vi "pigeon_ver4_1.vi"() -> ()   [LabVIEW 2017]
uses:
  <vilib>/eio/EIONode/EIONode.xnode
  <vilib>/Platform/TimedLoop/XDataNode/XDataNode.xnode
  <vilib>/Platform/TimedLoop/XDataNode/nitl_modes.ctl
  <vilib>/Platform/TimedLoop/XDataNode/XDNodeRunTimeDep.lvlib
  <vilib>/Platform/TimedLoop/XDataNode/wakeup.ctl
  <vilib>/Platform/TimedLoop/XDataNode/timing_clust.ctl
  <vilib>/rvi/DataTransferAndStorage/Container/XNode/niFpgaContainer.xnode
  <vilib>/rvi/eio/common/nirviEmuTemplateMethod_errors.vi
  <vilib>/rvi/Memory/Memory_Emulation/nirvimemoryFastEmulation.vi
  <vilib>/rvi/Memory/Memory_Emulation/nirvimemoryEmulation.vi
  <vilib>/rvi/interface/RandomDataEmulation/nirviRandomDataFpgaReadWriteTemplate.vi
  <vilib>/rvi/Analysis/common/FxpNativeNode/niFpgaFxpNative.xnode
panel:
  out "ramp loop end?":bool=TRUE
  out "ctr":i16
  out "ramp start val":fxp<+,15,15>
  out "Numeric":i16
  in  "analog ramp on":bool
  out "AI2":i16
  in  "Tab Control":enum32{"pigeon"}(tab)
  in  "AO7_pigeon":i16
  in  "AO7":i16
  in  "AO6":i16
  out "trigger AI1":bool
  in  "Tab Control 2":T1(tab)
  in  "square wave  on?":bool
  in  "square wave period":i32
  in  "IGBTswitch":bool caption="IGBT Switch circular"
  in  "Manual Override":bool
  in  "circular coil current":i16(slide) scale=0.0..32768.0
  in  "analog ramp period":i16
  in  "AO4":bool
  in  "analog wave shape":i16(ring) items=["Triangle", "Sawtooth", "Sin", ""]
  in  "analog ramp on  2":bool
  in  "End Current":fxp<+,16,16>
  out "approx rise time [uSec]":u32
  in  "Update Period (uSec)":u32=500
  in  "Points to Add (2^n - 1)":i16=3
  out "FIFO size":i16
  in  "AO0":i16
  in  "AO1":i16
  in  "AO2":i16
  in  "Run program":bool
  in  "halt processor":bool
  out "control flags":i8 format="%b"
  in  "host operation":i16
  in  "address":u16
  in  "data1":u16
  in  "data2":i32
  in  "repeat program":i32
  out "IP address":i16
  out "PMT1":i16=-4740
  out "ReA":i32
  out "RegB":i16
  out "RegC":i16
  out "exttrigger":bool=TRUE
  out "AI1":i16=161
  out "RegD":i16
  in  "AO4":i16
  in  "AO3":i16
  out "Connector0/AI0":i16
  in  "AO5":i16
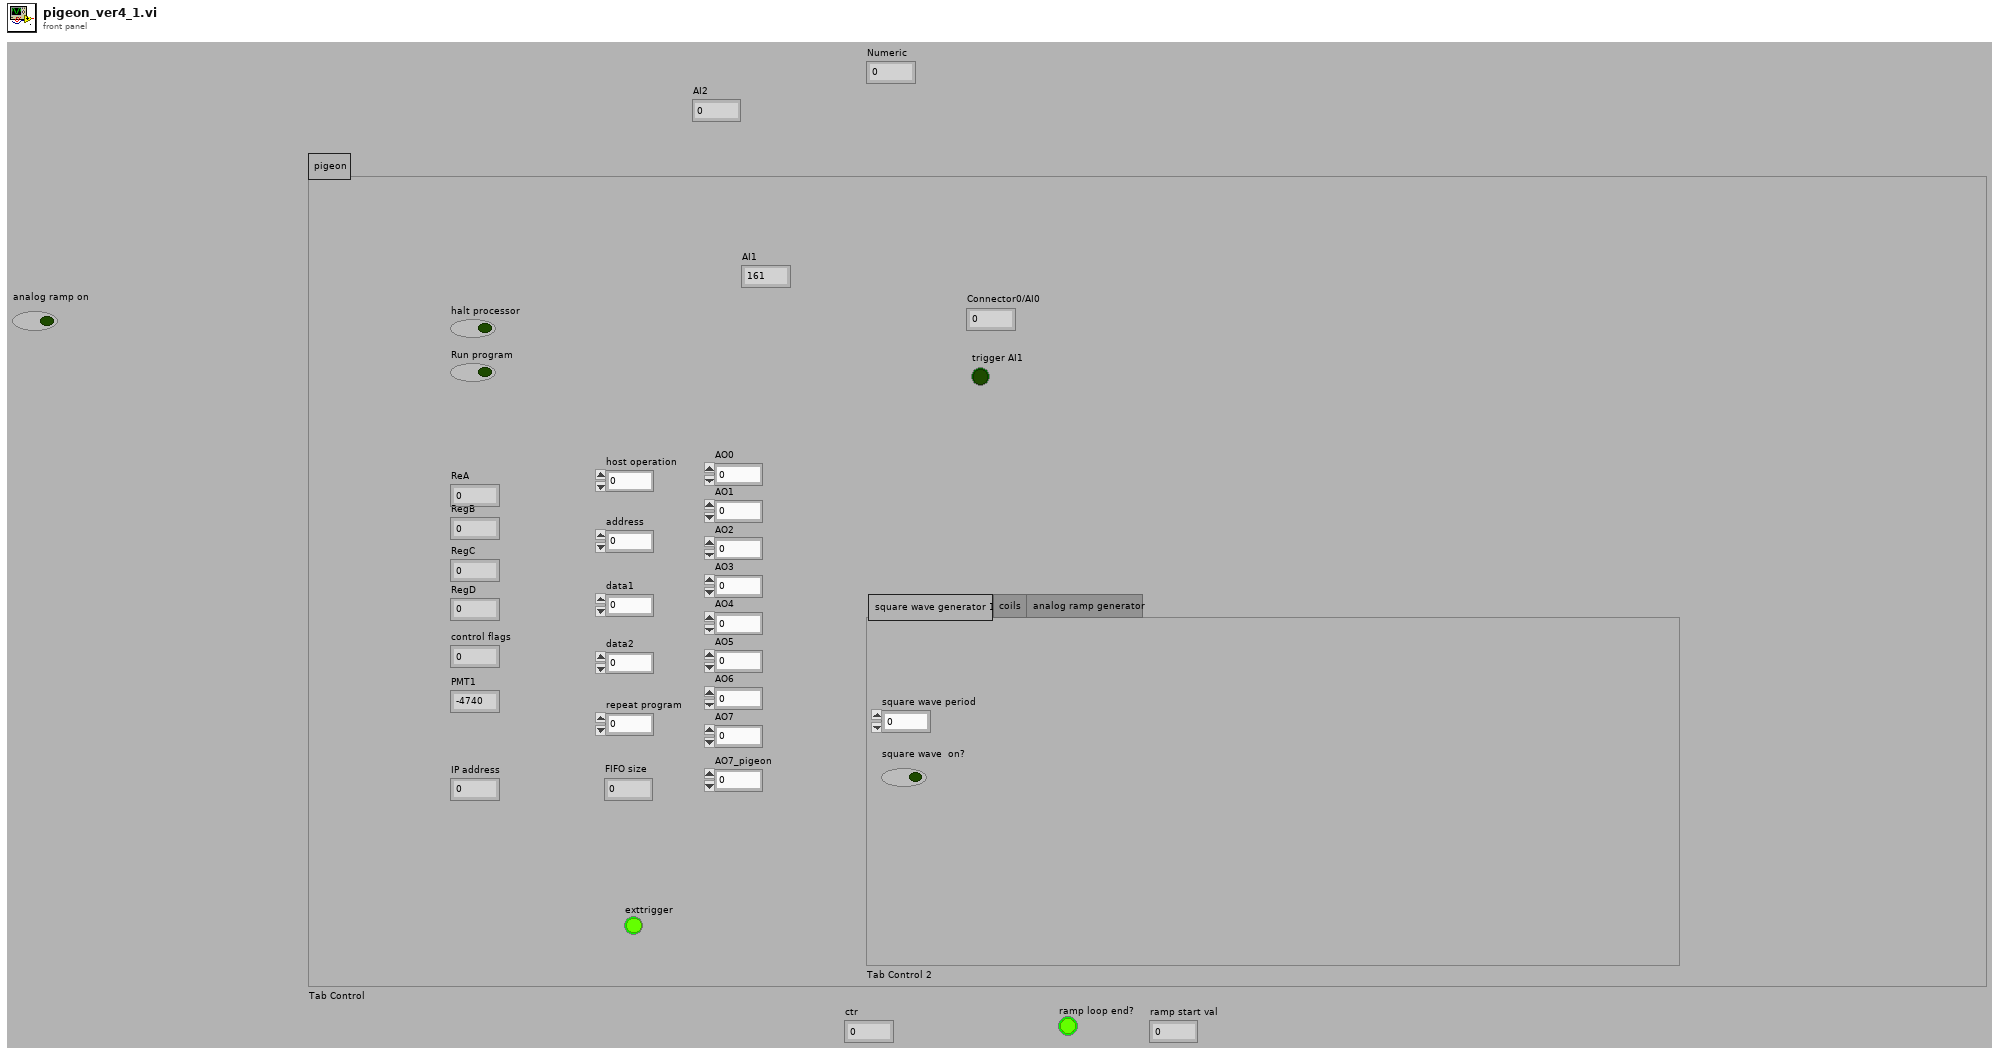
[diagram p1: front panel]
types:
  T1 = enum32{"square wave generator 1", "coils", "analog ramp generator"}
  T2 = typedef "XDNodeRunTimeDep.lvlib/timing_clust.ctl" = cluster{"Expected End [f-1]":u64, "Actual End [f-1]":u64, "Finished Late? [f-1]":bool, "Expected End [i-1]":u64, "Actual End [i-1]":u64, "Finished Late? [i-1]":bool, "Expected Start [i]":u64, "Actual Start [i]":u64, "Expected Start [f]":u64, "Actual Start [f]":u64, "Source Name":string, "Structure Name":string, "Period":i64, "Deadline":i64, "Offset":i64, "Start":i64, "Priority":i32, "Timeout":i32, "Mode":T3, "Wakeup Reason":T4, "Error":errorcluster, "Source Type":string, "Secondary Source Type":string, "Global End Time":u64, "Global Start Time":u64, "Frame Duration":u64, "Iteration Duration":u64, "Assigned CPU":i32, "I/O Scan Engine Mode":u32}
  T3 = typedef "XDNodeRunTimeDep.lvlib/nitl_modes.ctl" = enum32{"No Change", "Process missed periods, maintain original phase", "Discard missed periods, maintain original phase", "Process missed periods, ignore original phase", "Discard missed periods, ignore original phase"}
  T4 = typedef "XDNodeRunTimeDep.lvlib/wakeup.ctl" = enum32{"Normal", "Aborted", "Asynchronous wakeup", "Timing source error", "Timed loop error", "Timeout"}
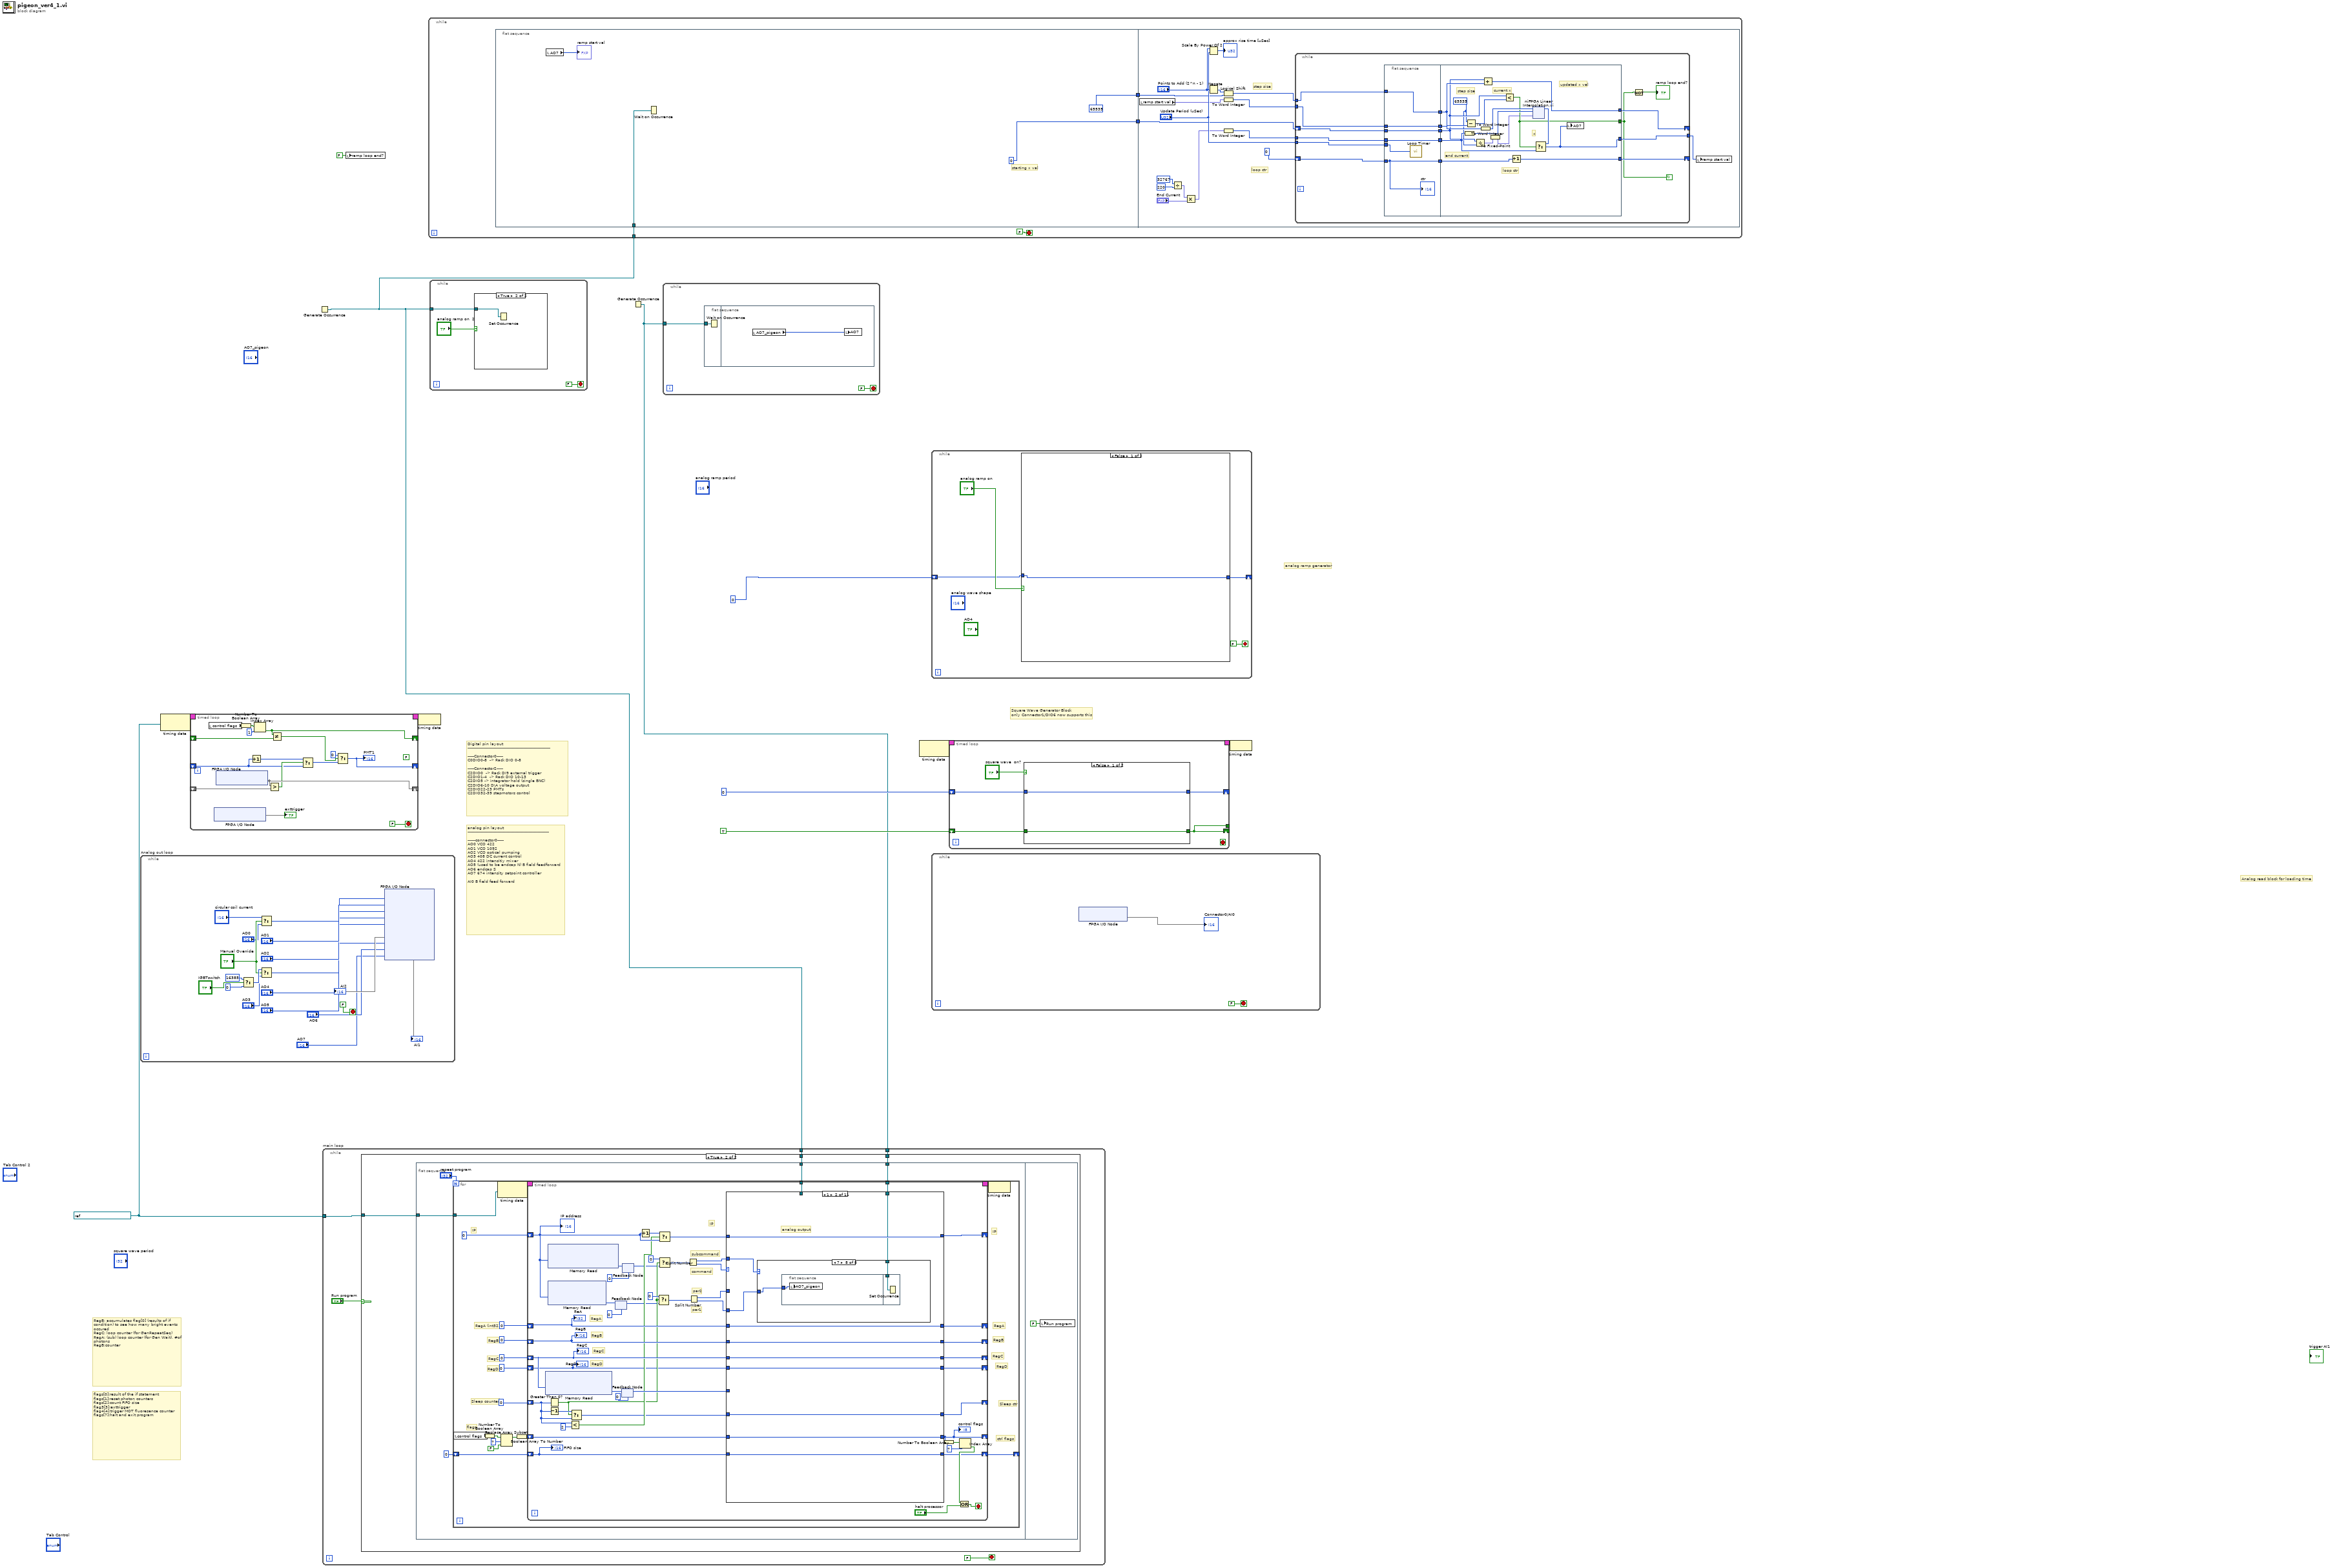
[diagram p0: block diagram]
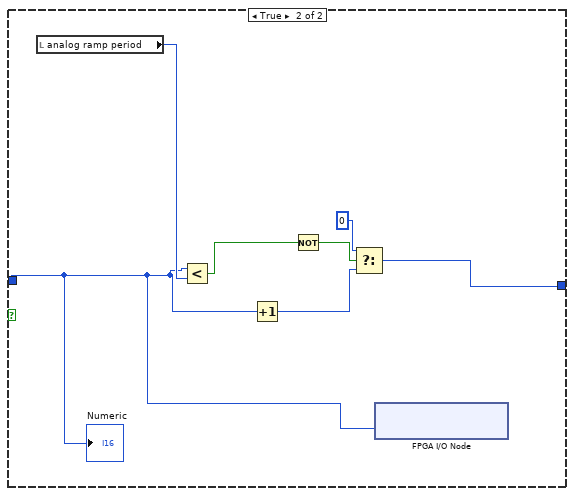
[diagram p3: hidden frame]
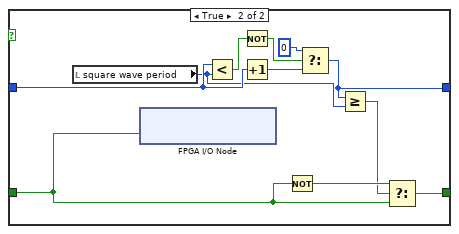
[diagram p4: hidden frame]
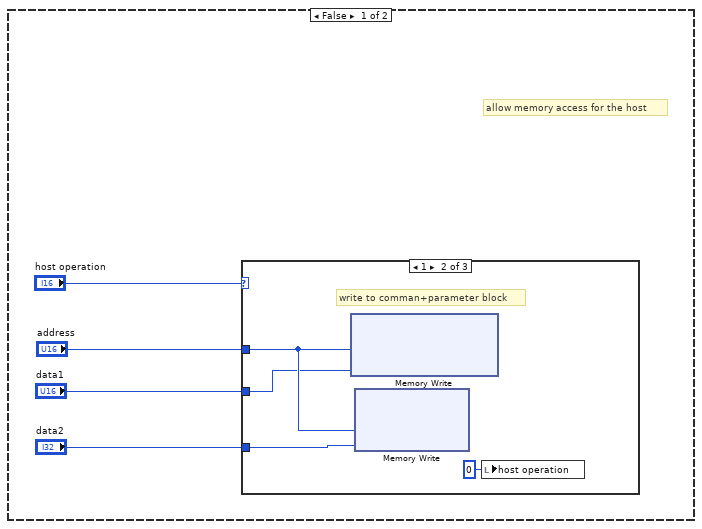
[diagram p5: hidden frame]
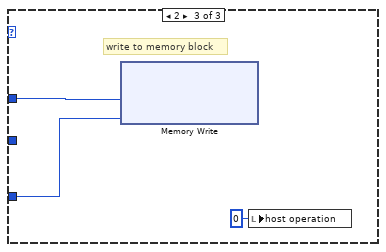
[diagram p7: hidden frame]
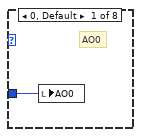
[diagram p9: hidden frame]
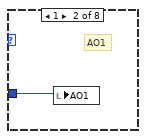
[diagram p10: hidden frame]
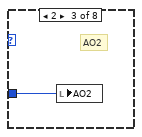
[diagram p11: hidden frame]
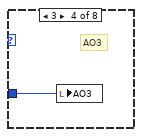
[diagram p12: hidden frame]
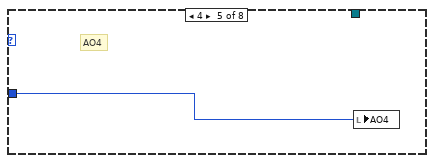
[diagram p13: hidden frame]
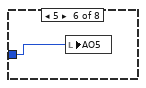
[diagram p14: hidden frame]
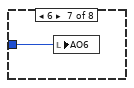
[diagram p15: hidden frame]
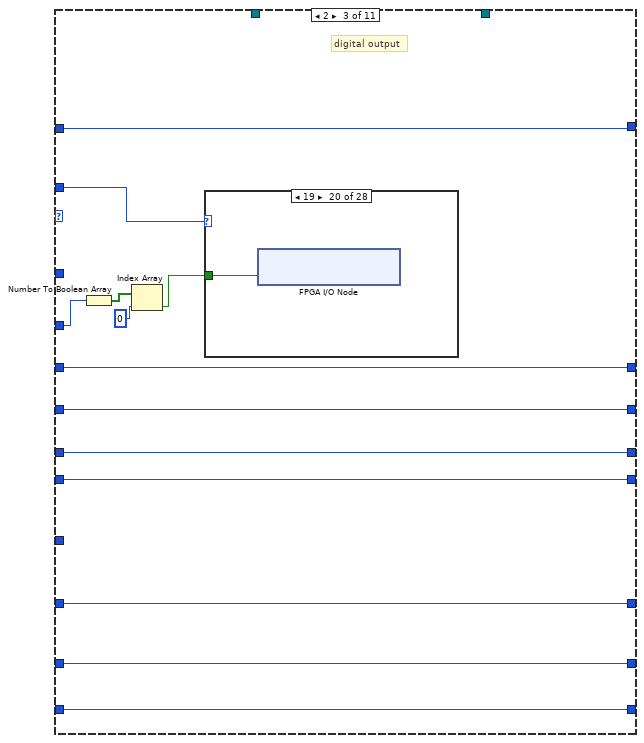
[diagram p16: hidden frame]
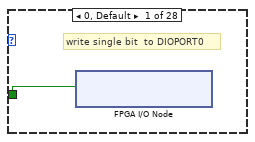
[diagram p17: hidden frame]
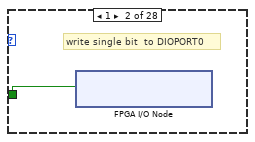
[diagram p18: hidden frame]
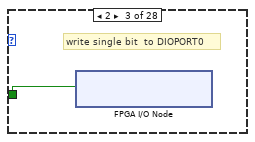
[diagram p19: hidden frame]
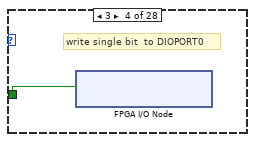
[diagram p20: hidden frame]
diagram:
  w9 = refnum<k21> "40 MHz Onboard Clock" ("FPGA Clock")
  # "analog ramp generator"
  # "Analog read block for loading time"
  # "Square Wave Generator Block\nonly Connector1/DIO6 now supports this"
  # "RegB: accumulates flag[0] (results of if condition) to see how many bright events occured\nRegC: loop counter (for GenRepeatSeq)\nRegA: (sub) loop counter (for Gen Wait), #of     photons \nRegB:counter"
  # "flags[0]:result of the if statement\nflags[1]:reset photon counters\nflags[2]:count FIFO size\nflag3[3]:exttrigger\nflag4[4]:trigger MOT fluoresence counter\nflags[7]:halt and exit program"
  # "Digital pin layout\n----------------------------------------------------------------\n\n-----Connector0-----\nC0DIO0-8  -> Rack DIO 0-8\n\n-----Connector2-----\nC2DIO0  -> Rack DI9 external trigger \nC2DIO1-4  -> Rack DIO 10-13\nC2DIO5 -> integrator hold (single BNC)\nC2DIO6-10 D\\A voltage output\nC2DIO22-23 PMTs\nC2DIO32-39 stepmotors control"
  # "analog pin layout\n---------------------------------------------------------------\n\n------connector0-----\nAO0 VCO 422\nAO1 VCO 1092\nAO2 VCO optical pumping\nAO3 408 DC current control\nAO4 422 intensitiy mixer\nAO5 (used to be endcap N) B field feedforward\nAO6 endcap S\nAO7 674 intensity setpoint controller\n\nAI0 B field feed forward"
  n1 = while "Analog out loop" {
    stop <- FALSE stop-if-true
    n2 = Select(t=i16 16385, s="IGBTswitch", f=i16 0) -> (s? t:f=w20:i16)
    n3 = Select(t="circular coil current", s="Manual Override", f="AO0") -> (s? t:f=w14:i16)
    n4 = Select(t=w20, s="Manual Override", f="AO3") -> (s? t:f=w19:i16)
    n5 = xnode "FPGA I/O Node"("Connector0/AO0"=w14, "Connector0/AO1"="AO1", "Connector0/AO2"="AO2", "Connector0/AO3"=w19, "Connector0/AO4"="AO4", "Connector0/AO5"="AO5", "Connector0/AO6"="AO6", "Connector0/AO7"="AO7") -> ("Connector0/AI1"=→"AI1", "Connector0/AI2"=→"AI2")  [unwired: 10 in, 10 out]
  }
  n6 = node-c288(w9) -> (w11:T2)
  n7 = timed-loop {
    timing: w11 -> [_]
    timing-out: [_] -> w10
    shift-right: [w44] -> _
    shift-left: _ -> [w33]
    shift-right: [w37] -> _
    shift-left: _ -> [w46]
    shift-right: [w39] -> _
    shift-left: _ -> [w40]
    stop <- FALSE stop-if-true
    (unwired) FALSE
    n8 = local read "control flags"() -> (w41:i8)
    n9 = xnode "FPGA I/O Node"() -> ("Connector2/DIO0"=→"exttrigger")  [unwired: 1 in, 1 out]
    n10 = xnode "FPGA I/O Node"() -> ("Connector0/DIO0"=w37)  [unwired: 1 in, 1 out]
    n11 = Number To Boolean Array(number=w41) -> (Boolean array=w42:bool[])
    n12 = Increment(x=w33) -> (x+1=w34:u16)
    n13 = Index Array(array=w42, index=1) -> (element=w39:bool)
    n14 = Greater?(x=w37, y=w46) -> (0:w36:bool)
    n15 = Not Equal?(x=w39, y=w40) -> (x != y?=w31:bool)
    n16 = Select(t=w34, s=w36, f=w33) -> (s? t:f=w45:u16)
    n17 = Select(t=u16 0, s=w31, f=w45) -> (s? t:f=w44:u16)
    "PMT1" <- w44
  }
  n18 = Generate Occurrence() -> (w2:refnum<k4>)
  n19 = local write "ramp loop end?"(FALSE ("ramp loop end?")) -> ()
  n20 = node-c288(w10) -> ()
  n21 = while {
    tunnel: w2 -> [w49]
    stop <- FALSE stop-if-true
    n22 = flat-sequence {
      tunnel: [u16 0] -> w51
      tunnel: [u16 65535 ("x")] -> w50
      tunnel: w49 -> [w53]
      tunnel: w51 -> [w61]
      tunnel: w50 -> [w62]
      frame #0 {
        # "starting x val"
        n23 = local read "AO7"() -> (→"ramp start val":i16)
        n24 = Wait on Occurrence(2:w53) -> ()  [unwired: 2 in, 1 out]
      }
      frame #1 {
        # "loop ctr"
        # "step size"
        n25 = local read "ramp start val"() -> (w58:fxp<+,15,15>)
        n26 = Divide(x=i16 32767, y=i16 220) -> (x/y=w71:fxp<+,16,16>)
        n27 = Multiply(x=w71, y="End Current") -> (x*y=w59:fxp<+,32,32>)
        n28 = Scale By Power Of 2(n="Points to Add (2^n - 1)", x="Update Period (uSec)") -> (x*2^n=→"approx rise time [uSec]":u32)
        n29 = Negate(x="Points to Add (2^n - 1)") -> (-x=w66:i16)
        n30 = Logical Shift(y=w66, x=w62) -> (x << y=w67:u16)
        n31 = To Word Integer(number=w58) -> (16bit integer=w69:i16)
        n32 = To Word Integer(number=w59) -> (16bit integer=w68:i16)
        n33 = while {
          tunnel: w67 -> [w77]
          tunnel: w69 -> [w89]
          tunnel: w68 -> [w88]
          shift-right: [w87] -> _
          shift-left: w61 -> [w76]
          tunnel: "Update Period (uSec)" -> [w86]
          shift-right: [w80] -> _
          shift-left: i16 0 -> [w78]
          tunnel: [w79] -> w60
          stop <- w75 continue-if-true
          n34 = flat-sequence {
            tunnel: w77 -> [w94]
            tunnel: [w94] -> w85
            tunnel: w89 -> [w93]
            tunnel: [w93] -> w84
            tunnel: w88 -> [w92]
            tunnel: [w92] -> w83
            tunnel: w76 -> [w91]
            tunnel: [w91] -> w82
            tunnel: w86 -> [w95]
            tunnel: w78 -> [w90]
            tunnel: [w90] -> w81
            tunnel: w85 -> [w103]
            tunnel: w84 -> [w111]
            tunnel: w83 -> [w101]
            tunnel: w82 -> [w99]
            tunnel: [w104] -> w75
            tunnel: [w105] -> w87
            tunnel: [w107] -> w80
            tunnel: w81 -> [w106]
            tunnel: [w96] -> w79
            frame #0 {
              n35 = call "Loop Timer"("Count(uSec)"=w95) -> ()  [unwired: 1 out]
              "ctr" <- w90
            }
            frame #1 {
              w97 = u16 65535 ("x")
              # "current x"
              # "end current"
              # "x"
              # "loop ctr"
              # "updated x val"
              # "step size"
              n36 = To Word Integer(number=w101) -> (16bit integer=w108:i16)
              n37 = Subtract(x=w97, y=w103) -> (x-y=w102:u16)
              n38 = Divide(x=w99, y=w97) -> (x/y=w98:fxp<+,16,0>)
              n39 = To Word Integer(number=w111) -> (16bit integer=w109:i16)
              n40 = Add(x=w99, y=w103) -> (x+y=w105:u16)
              n41 = To Fixed-Point(number=w98) -> (fixed-point=w100:fxp<+,16,0>)  [unwired: 1 in]
              n42 = Less?(x=w99, y=w102) -> (x < y?=w104:bool)
              n43 = Increment(x=w106) -> (x+1=w107:i16)
              n44 = xnode ("niFPGA Linear Interpolation.vi")("y0"=w109, "y1"=w108, "x"=w100) -> ("y"=w110:i16)
              n45 = Select(t=w110, s=w104, f=w101) -> (s? t:f=w96:i16)
              n46 = local write "AO7"(w96) -> ()
            }
          }
          n47 = Not(x=w75) -> (.not. x?=→"ramp loop end?":bool)
        }
        n48 = local write "ramp start val"(w60) -> ()
      }
    }
  }
  n49 = while {
    tunnel: w2 -> [w124]
    stop <- FALSE stop-if-true
    n50 = case shown="True" "analog ramp on  2" {
      tunnel: w124 -> [_ w126]
      frame False {
      }
      frame True {
        n51 = Set Occurrence(w126) -> ()
      }
    }
  }
  n52 = Generate Occurrence() -> (w1:refnum<k4>)
  n53 = while "main loop" {
    tunnel: w9 -> [w129]
    tunnel: w2 -> [w128]
    tunnel: w1 -> [w127]
    stop <- FALSE ("stop") stop-if-true
    n54 = case shown="True" "Run program" {
      tunnel: w129 -> [_ w145]
      tunnel: w128 -> [_ w144]
      tunnel: w127 -> [_ w143]
      frame False {
        # "allow memory access for the host"
        n55 = case shown="1" "host operation" {
          tunnel: "address" -> [_ w137 w142]
          tunnel: "data1" -> [_ w136 _]
          tunnel: "data2" -> [_ w139 w140]
          frame 0, Default {
          }
          frame 1 {
            # "write to comman+parameter block"
            n56 = xnode ("Memory Write")("Address"=w137, "Data"=w136) -> ()  [unwired: 1 in, 1 out]
            n57 = xnode ("Memory Write")("Address"=w137, "Data"=w139) -> ()  [unwired: 1 in, 1 out]
            n58 = local write "host operation"(i16 0 ("host operation")) -> ()
          }
          frame 2 {
            # "write to memory block"
            n59 = xnode ("Memory Write")("Address"=w142, "Data"=w140) -> ()  [unwired: 1 in, 1 out]
            n60 = local write "host operation"(i16 0 ("host operation")) -> ()
          }
        }
      }
      frame True {
        n61 = flat-sequence {
          tunnel: w145 -> [w149]
          tunnel: w144 -> [w147]
          tunnel: w143 -> [w146]
          frame #0 {
            n62 = for {
              N: "repeat program" -> [_]
              tunnel: w149 -> [w163]
              shift-right: [w154] -> _
              shift-left: i16 0 -> [w155]
              tunnel: w147 -> [w152]
              tunnel: w146 -> [w151]
              # "ctrl flags"
              # "Sleep ctr"
              # "RegD"
              # "RegD"
              # "Sleep counter"
              # "flags"
              # "RegC"
              # "RegB"
              # "RegA"
              # "RegC"
              # "RegB"
              # "RegA (int32)"
              # "IP"
              # "IP"
              n63 = local read "control flags"() -> (w158:i8)
              n64 = Number To Boolean Array(number=w158) -> (Boolean array=w162:bool[])
              n65 = node-c288(w163) -> (w169:T2)
              n66 = Replace Array Subset(array=w162, new element=FALSE ("new element/subarray"), index=7) -> (w160:bool[])
              n67 = Boolean Array To Number(Boolean array=w160) -> (number=w161:u8)
              n68 = timed-loop {
                timing: w169 -> [_]
                timing-out: [_] -> w168
                shift-right: [w206] -> _
                shift-left: i16 0 -> [w189]
                shift-right: [w202] -> _
                shift-left: 0 -> [w198]
                shift-right: [w214] -> _
                shift-left: i16 0 -> [w205]
                shift-right: [w213] -> _
                shift-left: i16 0 -> [w197]
                shift-right: [w203] -> _
                shift-left: w161 -> [w204]
                shift-right: [w196] -> _
                shift-left: i16 0 -> [w187]
                shift-right: [w178] -> w154
                shift-left: w155 -> [w177]
                shift-right: [w175] -> _
                shift-left: i16 0 -> [w176]
                tunnel: w152 -> [w171]
                tunnel: w151 -> [w170]
                stop <- w209 stop-if-true
                # "RegD"
                # "IP"
                # "RegC"
                # "RegB"
                # "RegA"
                # "par1"
                # "par2"
                # "subcommand"
                # "command"
                n69 = xnode ("Memory Read")("Address"=w197) -> ("Data"=w201:i16)  [unwired: 2 in, 2 out]
                n70 = xnode ("Memory Read")("Address"=w189) -> ("Data"=w184:u16)  [unwired: 1 in, 1 out]
                n71 = xnode ("Memory Read")("Address"=w189) -> ("Data"=w180:i32)  [unwired: 1 in, 1 out]
                n72 = Greater Than 0?(x=w187) -> (x > 0?=w182:bool)
                n73 = Decrement(x=w187) -> (x-1=w188:u32)
                n74 = Less?(x=w187, y=u32 2) -> (x < y?=w186:bool)
                n75 = Select(t=w188, s=w182, f=w187) -> (s? t:f=w185:u32)
                n76 = feedback-in #1(w180) -> ()
                n77 = feedback #1(u32 0 ("Data")) -> (w179:u32)
                n78 = feedback-in #2(w201) -> ()
                n79 = feedback #2(0) -> (w200:i32)
                n80 = feedback-in #3(w184) -> ()
                n81 = feedback #3(u16 0 ("Data")) -> (w181:u16)
                n82 = Increment(x=w189) -> (x+1=w190:u16)
                n83 = Select(t=0, s=w182, f=w179) -> (s? t:f=w193:u32)
                n84 = Select(t=w190, s=w186, f=w189) -> (s? t:f=w195:u16)
                n85 = Select(t=u16 0, s=w182, f=w181) -> (s? t:f=w194:u16)
                n86 = Split Number(x=w194) -> (hi(x)=w215:u8, lo(x)=w216:u8)
                n87 = Split Number(x=w193) -> (hi(x)=w207:u16, lo(x)=w208:u16)
                n88 = case shown="1" w216 {
                  tunnel: w208 -> [_ w234 w251 _ w331 w451 w525 _ _ w585 _]
                  tunnel: w207 -> [_ _ _ _ w324 w450 w524 _ _ w586 _]
                  tunnel: w215 -> [_ w235 w259 w298 w332 w455 _ w543 _ w567 _]
                  tunnel: w198 -> [w224 w233 w258 w290 w330 w452 w529 w547 w563 w584 w614]
                  tunnel: [w224 w233 w258 w290 w327 w452 w529 w547 w563 w583 w614] -> w202
                  tunnel: w205 -> [w223 w232 w257 w289 w329 w453 w530 w546 w566 w582 w615]
                  tunnel: w197 -> [w222 w231 w256 w296 w328 w454 w531 w545 w565 w580 w616]
                  tunnel: [w223 w232 w257 w288 w326 w453 w530 w546 w566 w581 w615] -> w214
                  tunnel: [w222 w231 w256 w296 w325 w454 w531 w545 w565 w579 w616] -> w213
                  tunnel: [w220 w230 w255 w297 w320 w458 w523 w549 w564 w569 w613] -> w206
                  tunnel: w195 -> [w220 w230 w255 w297 w321 w458 _ w549 w564 w570 w613]
                  tunnel: [w221 w229 w254 w294 w322 w457 w522 w538 w560 w573 w619] -> w203
                  tunnel: w204 -> [w221 w229 w254 w295 w323 w456 w522 w537 w559 w574 w619]
                  tunnel: w200 -> [_ _ _ _ w314 w449 _ _ _ _ _]
                  tunnel: w185 -> [w219 w228 w249 w293 w319 w448 w521 w535 w556 w576 w620]
                  tunnel: [w219 w228 w249 w293 w318 w448 w521 w535 w556 w575 w620] -> w196
                  tunnel: w177 -> [w218 w227 w248 w292 w317 w447 w520 w534 w555 w571 w618]
                  tunnel: [w218 w227 w248 w292 w317 w447 w520 w533 w555 w572 w618] -> w178
                  tunnel: w176 -> [w217 w226 w247 w291 w316 w446 w519 w532 w554 w578 w617]
                  tunnel: [w217 w226 w247 w291 w315 w446 w519 w532 w554 w577 w617] -> w175
                  tunnel: w171 -> [_ _ _ _ _ _ _ _ _ w568 _]
                  tunnel: w170 -> [_ w225 _ _ _ _ _ _ _ _ _]
                  frame 0, Default {
                  }
                  frame 1 {
                    # "analog output"
                    n89 = case shown="7" w235 {
                      tunnel: w234 -> [w236 w237 w238 w239 w240 w241 w242 w244]
                      tunnel: w225 -> [_ _ _ _ _ _ _ w243]
                      frame 0, Default {
                        # "AO0"
                        n90 = local write "AO0"(w236) -> ()
                      }
                      frame 1 {
                        # "AO1"
                        n91 = local write "AO1"(w237) -> ()
                      }
                      frame 2 {
                        # "AO2"
                        n92 = local write "AO2"(w238) -> ()
                      }
                      frame 3 {
                        # "AO3"
                        n93 = local write "AO3"(w239) -> ()
                      }
                      frame 4 {
                        # "AO4"
                        n94 = local write "AO4"(w240) -> ()
                      }
                      frame 5 {
                        n95 = local write "AO5"(w241) -> ()
                      }
                      frame 6 {
                        n96 = local write "AO6"(w242) -> ()
                      }
                      frame 7 {
                        n97 = flat-sequence {
                          tunnel: w244 -> [w245]
                          tunnel: w243 -> [w246]
                          frame #0 {
                            n98 = local write "AO7_pigeon"(w245) -> ()
                          }
                          frame #1 {
                            n99 = Set Occurrence(w246) -> ()
                          }
                        }
                      }
                    }
                  }
                  frame 2 {
                    # "digital output"
                    n100 = Number To Boolean Array(number=w251) -> (Boolean array=w252:bool[])
                    n101 = Index Array(array=w252, index=0) -> (element=w250:bool)
                    n102 = case shown="19" w259 {
                      tunnel: w250 -> [w260 w261 w262 w263 w264 w265 w266 w267 w268 w269 w270 w271 w272 w273 w274 w275 w276 w277 w278 w279 w280 w281 w282 w283 w284 w285 w286 w287]
                      frame 0, Default {
                        # "write single bit  to DIOPORT0"
                        n103 = xnode "FPGA I/O Node"("Connector1/DIO0"=w260) -> ()  [unwired: 1 in, 1 out]
                      }
                      frame 1 {
                        # "write single bit  to DIOPORT0"
                        n104 = xnode "FPGA I/O Node"("Connector1/DIO1"=w261) -> ()  [unwired: 1 in, 1 out]
                      }
                      frame 2 {
                        # "write single bit  to DIOPORT0"
                        n105 = xnode "FPGA I/O Node"("Connector1/DIO2"=w262) -> ()  [unwired: 1 in, 1 out]
                      }
                      frame 3 {
                        # "write single bit  to DIOPORT0"
                        n106 = xnode "FPGA I/O Node"("Connector1/DIO3"=w263) -> ()  [unwired: 1 in, 1 out]
                      }
                      frame 4 {
                        # "write single bit  to DIOPORT0"
                        n107 = xnode "FPGA I/O Node"("Connector1/DIO4"=w264) -> ()  [unwired: 1 in, 1 out]
                      }
                      frame 5 {
                        # "write single bit  to DIOPORT0"
                        n108 = xnode "FPGA I/O Node"("Connector1/DIO5"=w265) -> ()  [unwired: 1 in, 1 out]
                      }
                      frame 6 {
                        # "write single bit  to DIOPORT0"
                        n109 = xnode "FPGA I/O Node"("Connector1/DIO6"=w266) -> ()  [unwired: 1 in, 1 out]
                      }
                      frame 7 {
                        # "write single bit  to DIOPORT0"
                        n110 = xnode "FPGA I/O Node"("Connector1/DIO7"=w267) -> ()  [unwired: 1 in, 1 out]
                      }
                      frame 8 {
                        # "write single bit  to DIOPORT0"
                        n111 = xnode "FPGA I/O Node"("Connector1/DIO8"=w268) -> ()  [unwired: 1 in, 1 out]
                      }
                      frame 9 {
                        n112 = xnode "FPGA I/O Node"("Connector1/DIO9"=w269) -> ()  [unwired: 1 in, 1 out]
                      }
                      frame 10 {
                        n113 = xnode "FPGA I/O Node"("Connector1/DIO10"=w270) -> ()  [unwired: 1 in, 1 out]
                      }
                      frame 11 {
                        n114 = xnode "FPGA I/O Node"("Connector1/DIO11"=w271) -> ()  [unwired: 1 in, 1 out]
                      }
                      frame 12 {
                        n115 = xnode "FPGA I/O Node"("Connector1/DIO12"=w272) -> ()  [unwired: 1 in, 1 out]
                      }
                      frame 13 {
                        n116 = xnode "FPGA I/O Node"("Connector1/DIO13"=w273) -> ()  [unwired: 1 in, 1 out]
                      }
                      frame 14 {
                        n117 = xnode "FPGA I/O Node"("Connector1/DIO14"=w274) -> ()  [unwired: 1 in, 1 out]
                      }
                      frame 15 {
                        n118 = xnode "FPGA I/O Node"("Connector1/DIO15"=w275) -> ()  [unwired: 1 in, 1 out]
                      }
                      frame 16 {
                        n119 = xnode "FPGA I/O Node"("Connector1/DIO16"=w276) -> ()  [unwired: 1 in, 1 out]
                      }
                      frame 17 {
                        n120 = xnode "FPGA I/O Node"("Connector1/DIO17"=w277) -> ()  [unwired: 1 in, 1 out]
                      }
                      frame 18 {
                        n121 = xnode "FPGA I/O Node"("Connector1/DIO18"=w278) -> ()  [unwired: 1 in, 1 out]
                      }
                      frame 19 {
                        n122 = xnode "FPGA I/O Node"("Connector1/DIO19"=w279) -> ()  [unwired: 1 in, 1 out]
                      }
                      frame 20 {
                        n123 = xnode "FPGA I/O Node"("Connector2/DIO12"=w280) -> ()  [unwired: 1 in, 1 out]
                      }
                      frame 21 {
                        n124 = xnode "FPGA I/O Node"("Connector2/DIO17"=w281) -> ()  [unwired: 1 in, 1 out]
                      }
                      frame 22 {
                        n125 = xnode "FPGA I/O Node"("Connector2/DIO19"=w282) -> ()  [unwired: 1 in, 1 out]
                      }
                      frame 23 {
                        n126 = xnode "FPGA I/O Node"("Connector2/DIO18"=w283) -> ()  [unwired: 1 in, 1 out]
                      }
                      frame 24 {
                        n127 = xnode "FPGA I/O Node"("Connector2/DIO21"=w284) -> ()  [unwired: 1 in, 1 out]
                      }
                      frame 25 {
                        n128 = xnode "FPGA I/O Node"("Connector2/DIO24"=w285) -> ()  [unwired: 1 in, 1 out]
                      }
                      frame 26 {
                        n129 = xnode "FPGA I/O Node"("Connector2/DIO25"=w286) -> ()  [unwired: 1 in, 1 out]
                      }
                      frame 27 {
                        n130 = xnode "FPGA I/O Node"("Connector2/DIO20"=w287) -> ()  [unwired: 1 in, 1 out]
                      }
                    }
                  }
                  frame 3 {
                    # "photon counting"
                    n131 = case shown="3" w298 {
                      tunnel: [w299 w301 w313] -> w288
                      tunnel: w289 -> [w299 w302 w313]
                      tunnel: w295 -> [w300 w304 w311]
                      tunnel: [w300 w304 w310] -> w294
                      frame 2, Default {
                      }
                      frame 1 {
                        # "PMT1"
                        n132 = local read "PMT1"() -> (w303:i16)
                        n133 = Add(x=w303, y=w302) -> (x+y=w301:u16)
                      }
                      frame 3 {
                        # "Reset  photon counter"
                        # "make a Not gate of flag(1)"
                        n134 = Number To Boolean Array(number=w311) -> (Boolean array=w308:bool[])
                        n135 = Index Array(array=w308, index=1) -> (element=w306:bool)
                        n136 = Not(x=w306) -> (.not. x?=w305:bool)
                        n137 = Replace Array Subset(array=w308, new element=w305, index=1) -> (w309:bool[])
                        n138 = Boolean Array To Number(Boolean array=w309) -> (number=w310:u8)
                      }
                    }
                  }
                  frame 4 {
                    # "registers operation"
                    n139 = case shown="7" w332 {
                      tunnel: w331 -> [w338 w348 w355 _ _ _ _ w397 _ _ w424 w437]
                      tunnel: w330 -> [_ w347 w354 w361 w369 w377 w381 w402 w413 w419 w429 w442]
                      tunnel: w329 -> [w341 _ w353 w360 w371 w376 w389 w401 w412 w415 w427 w440]
                      tunnel: w328 -> [w340 w346 _ w363 w370 _ w382 w400 w411 w418 w428 w441]
                      tunnel: [w337 w347 w354 w361 w368 w377 w381 w402 w413 w419 w429 w442] -> w327
                      tunnel: [w341 w348 w353 w360 w371 w376 w388 w401 w412 w417 w427 w440] -> w326
                      tunnel: [w340 w346 w355 w362 w370 w376 w382 w400 w411 w418 w428 w441] -> w325
                      tunnel: w324 -> [w339 _ _ _ _ _ _ w398 _ _ _ w436]
                      tunnel: w323 -> [w336 w345 w352 w359 w367 w375 w383 w399 w410 w422 w432 w445]
                      tunnel: [w336 w345 w352 w359 w367 w375 w383 w399 w410 w422 w432 w445] -> w322
                      tunnel: w321 -> [w335 w344 w351 w358 w366 w374 w380 w391 w405 w421 w431 w444]
                      tunnel: [w335 w344 w351 w358 w366 w374 w380 w394 w408 w421 w431 w444] -> w320
                      tunnel: w319 -> [w334 w343 w350 w357 w365 w373 w379 _ _ w420 w430 w443]
                      tunnel: [w334 w343 w350 w357 w365 w373 w379 w395 w403 w420 w430 w443] -> w318
                      tunnel: w316 -> [w333 w342 w349 w356 w364 w372 w378 w390 w404 w414 _ w435]
                      tunnel: [w333 w342 w349 w356 w364 w372 w378 w390 w404 w414 w425 w434] -> w315
                      tunnel: w314 -> [_ _ _ _ _ _ _ _ w403 _ _ _]
                      frame 0, Default {
                        # "Set par1,2 to RegA"
                        n140 = Join Numbers(hi=w339, lo=w338) -> ((hi.lo)=w337:u32)
                      }
                      frame 1 {
                        # "Set par1 to RegB"
                      }
                      frame 2 {
                        # "Set par1 to RegC"
                      }
                      frame 3 {
                        # "increase RegC by 1"
                        n141 = Increment(x=w363) -> (x+1=w362:u16)
                      }
                      frame 4 {
                        # "increase RegA by 1"
                        n142 = Increment(x=w369) -> (x+1=w368:u32)
                      }
                      frame 5 {
                        # "Set regC to regB"
                      }
                      frame 6 {
                        # "regB<-regB+flags[0]"
                        n143 = Number To Boolean Array(number=w383) -> (Boolean array=w387:bool[])
                        n144 = Index Array(array=w387, index=0) -> (element=w385:bool)
                        n145 = Boolean To (0,1)(Boolean=w385) -> (0, 1=w384:i16)
                        n146 = Add(x=w384, y=w389) -> (x+y=w388:u16)
                      }
                      frame 7 {
                        # "Sleep counter = [par1 par2]"
                        n147 = Join Numbers(hi=w398, lo=w397) -> ((hi.lo)=w395:u32)
                        n148 = Greater?(x=w395, y=u32 0) -> (0:w393:bool)
                        n149 = Decrement(x=w391) -> (x-1=w392:u16)
                        n150 = Select(t=w392, s=w393, f=w391) -> (s? t:f=w394:u16)
                      }
                      frame 11 {
                        # "Sleep counter =par1* memory Block[RegC]"
                        n151 = Greater?(x=w403, y=u32 0) -> (0:w407:bool)
                        n152 = Decrement(x=w405) -> (x-1=w406:u16)
                        n153 = Select(t=w406, s=w407, f=w405) -> (s? t:f=w408:u16)
                      }
                      frame 8 {
                        # "RegB=RegB+ RegA(lo)"
                        n154 = Split Number(x=w419) -> (lo(x)=w416:u16)  [unwired: 1 out]
                        n155 = Add(x=w416, y=w415) -> (x+y=w417:u16)
                      }
                      frame 9 {
                        # "RegD<-AI1+par1"
                        n156 = To Word Integer(number=w424) -> (16bit integer=w423:i16)
                        n157 = local read "AI1"() -> (w426:i16)
                        n158 = Add(x=w423, y=w426) -> (x+y=w425:i16)
                      }
                      frame 10 {
                        # "RegD<-RegD*2^par1*par2"
                        n159 = To Word Integer(number=w436) -> (16bit integer=w438:i16)
                        n160 = To Word Integer(number=w437) -> (16bit integer=w439:i16)
                        n161 = Multiply(x=w438, y=w435) -> (x*y=w433:i16)
                        n162 = Scale By Power Of 2(n=w439, x=w433) -> (x*2^n=w434:i16)
                      }
                    }
                  }
                  frame 5 {
                    # "If statement"
                    n163 = case shown="4" w455 {
                      tunnel: [w468 w476 w484 w492 w502 w505 w513] -> w457
                      tunnel: w456 -> [w467 w475 w483 w491 w501 w506 w514]
                      tunnel: w450 -> [w461 _ _ _ _ _ _]
                      tunnel: w454 -> [_ _ w479 w486 _ _ _]
                      tunnel: w453 -> [_ w470 _ w485 _ _ _]
                      tunnel: w452 -> [w462 _ _ _ _ w503 w511]
                      tunnel: w451 -> [w460 w469 w478 _ _ w504 _]
                      tunnel: w449 -> [_ _ _ _ _ _ w518]
                      frame 0, Default {
                        # "The if regA =  [par1,par2]"
                        n164 = Number To Boolean Array(number=w467) -> (Boolean array=w465:bool[])
                        n165 = Join Numbers(hi=w461, lo=w460) -> ((hi.lo)=w459:u32)
                        n166 = Equal?(x=w459, y=w462) -> (x = y?=w463:bool)
                        n167 = Replace Array Subset(array=w465, new element=w463, index=0) -> (w464:bool[])
                        n168 = Boolean Array To Number(Boolean array=w464) -> (number=w468:u8)
                      }
                      frame 1 {
                        # "The if  regB >  par1"
                        n169 = Number To Boolean Array(number=w475) -> (Boolean array=w473:bool[])
                        n170 = Greater?(x=w470, y=w469) -> (0:w471:bool)
                        n171 = Replace Array Subset(array=w473, new element=w471, index=0) -> (w472:bool[])
                        n172 = Boolean Array To Number(Boolean array=w472) -> (number=w476:u8)
                      }
                      frame 2 {
                        # "The if  regC=  par1"
                        n173 = Number To Boolean Array(number=w483) -> (Boolean array=w481:bool[])
                        n174 = Equal?(x=w478, y=w479) -> (x = y?=w477:bool)
                        n175 = Replace Array Subset(array=w481, new element=w477, index=0) -> (w480:bool[])
                        n176 = Boolean Array To Number(Boolean array=w480) -> (number=w484:u8)
                      }
                      frame 3 {
                        # "The if  regB> regC"
                        n177 = Number To Boolean Array(number=w491) -> (Boolean array=w489:bool[])
                        n178 = Greater?(x=w485, y=w486) -> (0:w487:bool)
                        n179 = Replace Array Subset(array=w489, new element=w487, index=0) -> (w488:bool[])
                        n180 = Boolean Array To Number(Boolean array=w488) -> (number=w492:u8)
                      }
                      frame 4 {
                        w497 = 3 ("index")
                        # "external trigger rising edge"
                        n181 = Number To Boolean Array(number=w501) -> (Boolean array=w498:bool[])
                        n182 = local read "exttrigger"() -> (w494:bool)
                        n183 = Index Array(array=w498, index=w497) -> (element=w496:bool)
                        n184 = Not(x=w496) -> (.not. x?=w495:bool)
                        n185 = And(x=w494, y=w495) -> (x .and. y?=w493:bool)
                        n186 = Replace Array Subset(array=w498, new element #1=w493, index #1=0 ("index"), new element #2=w494, index #2=w497) -> (w499:bool[])
                        n187 = Boolean Array To Number(Boolean array=w499) -> (number=w502:u8)
                      }
                      frame 5 {
                        # "The if  regA >  par1"
                        n188 = Number To Boolean Array(number=w506) -> (Boolean array=w509:bool[])
                        n189 = Greater?(x=w503, y=w504) -> (0:w507:bool)
                        n190 = Replace Array Subset(array=w509, new element=w507, index=0) -> (w508:bool[])
                        n191 = Boolean Array To Number(Boolean array=w508) -> (number=w505:u8)
                      }
                      frame 6 {
                        # "The if  regA == memoryBlock(regC)"
                        n192 = Number To Boolean Array(number=w514) -> (Boolean array=w516:bool[])
                        n193 = Equal?(x=w511, y=w518) -> (x = y?=w512:bool)
                        n194 = Replace Array Subset(array=w516, new element=w512, index=0) -> (w515:bool[])
                        n195 = Boolean Array To Number(Boolean array=w515) -> (number=w513:u8)
                      }
                    }
                  }
                  frame 6 {
                    # "condition (flags[0]) goto\nuse par1=par2 for normal goto"
                    n196 = Number To Boolean Array(number=w522) -> (Boolean array=w528:bool[])
                    n197 = Index Array(array=w528, index=0) -> (element=w526:bool)
                    n198 = Select(t=w525, s=w526, f=w524) -> (s? t:f=w523:u16)
                  }
                  frame 7 {
                    w536 = 2 ("index")
                    # "make a Not gate of flag(2)"
                    # "push  to FIFO"
                    n199 = case shown="4" w543 {
                      tunnel: w547 -> [w550 _ _ _]
                      tunnel: w546 -> [_ w551 _ _]
                      tunnel: w545 -> [_ _ w552 _]
                      tunnel: [w550 w551 w552 w553] -> w544
                      frame 0, Default {
                        # "push RegA"
                      }
                      frame 1 {
                        # "push RegB"
                      }
                      frame 2 {
                        # "push RegC"
                      }
                      frame 4 {
                        n200 = local read "AI1"() -> (w553:i16)
                      }
                    }
                    n201 = Number To Boolean Array(number=w537) -> (Boolean array=w541:bool[])
                    n202 = Index Array(array=w541, index=w536) -> (element=w540:bool)
                    n203 = Not(x=w540) -> (.not. x?=w539:bool)
                    n204 = Replace Array Subset(array=w541, new element=w539, index=w536) -> (w542:bool[])
                    n205 = Increment(x=w534) -> (x+1=w533:i16)
                    n206 = Boolean Array To Number(Boolean array=w542) -> (number=w538:u8)
                    n207 = xnode ("FIFO Write")("Element"=w544, "Timeout"=0) -> ()  [unwired: 1 in, 2 out]
                  }
                  frame 8 {
                    # "Stop and reset program"
                    n208 = Number To Boolean Array(number=w559) -> (Boolean array=w562:bool[])
                    n209 = Replace Array Subset(array=w562, new element=TRUE ("new element/subarray"), index=7) -> (w561:bool[])
                    n210 = Boolean Array To Number(Boolean array=w561) -> (number=w560:u8)
                  }
                  frame 9 {
                    # "Cold Lab Specific instructions"
                    n211 = case shown="1" w567 {
                      tunnel: w586 -> [w599 w604]
                      tunnel: w585 -> [w598 w603]
                      tunnel: w584 -> [w595 w605]
                      tunnel: [w595 w605] -> w583
                      tunnel: w582 -> [w594 w606]
                      tunnel: [w594 w606] -> w581
                      tunnel: w580 -> [w593 w607]
                      tunnel: [w593 w607] -> w579
                      tunnel: w578 -> [w592 w608]
                      tunnel: [w592 w608] -> w577
                      tunnel: w576 -> [w591 w609]
                      tunnel: [w591 w609] -> w575
                      tunnel: w574 -> [w590 w610]
                      tunnel: [w590 w610] -> w573
                      tunnel: [w589 w611] -> w572
                      tunnel: w571 -> [w589 w611]
                      tunnel: w570 -> [w588 w602]
                      tunnel: [w588 w602] -> w569
                      tunnel: w568 -> [_ w601]
                      tunnel: w567 -> [w587 _]
                      frame 0, Default {
                        # "Run Square wave generator"
                        n212 = Greater?(x=w587, y=u8 0) -> (0:w596:bool)
                        n213 = Join Numbers(hi=w599, lo=w598) -> ((hi.lo)=w600:u32)
                        n214 = local write "square wave  on?"(w596) -> ()
                        n215 = local write "square wave period"(w600) -> ()
                      }
                      frame 1 {
                        # "start compression"
                        n216 = Set Occurrence(w601) -> ()
                        n217 = local write "Points to Add (2^n - 1)"(w603) -> ()
                        n218 = local write "End Current"(w604) -> ()
                      }
                    }
                  }
                  frame 10 {
                    n219 = local write "trigger AI1"(TRUE) -> ()
                  }
                }
                "control flags" <- w203
                n220 = Number To Boolean Array(number=w203) -> (Boolean array=w212:bool[])
                n221 = Index Array(array=w212, index=7) -> (element=w210:bool)
                n222 = Or(x=w210, y="halt processor") -> (x .or. y?=w209:bool)
                "IP address" <- w189
                "ReA" <- w198
                "RegB" <- w205
                "RegC" <- w197
                "FIFO size" <- w177
                "RegD" <- w176
              }
              n223 = node-c288(w168) -> ()
            }
          }
          frame #1 {
            n224 = local write "Run program"(FALSE ("Run program")) -> ()
          }
        }
      }
    }
  }
  n225 = while {
    tunnel: w1 -> [w629]
    stop <- FALSE stop-if-true
    n226 = flat-sequence {
      tunnel: w629 -> [w630]
      frame #0 {
        n227 = Wait on Occurrence(2:w630) -> ()  [unwired: 2 in, 1 out]
      }
      frame #1 {
        n228 = local read "AO7_pigeon"() -> (w631:i16)
        n229 = local write "AO7"(w631) -> ()
      }
    }
  }
  n230 = node-c288() -> (w8:T2)  [unwired: 1 in]
  n231 = while {
    shift-right: [w632] -> _
    shift-left: i16 0 -> [w633]
    stop <- FALSE stop-if-true
    n232 = case shown="False" "analog ramp on" {
      tunnel: [w636 w640] -> w632
      tunnel: w633 -> [w636 w637]
      frame False {
      }
      frame True {
        n233 = local read "analog ramp period"() -> (w639:i16)
        n234 = Less?(x=w637, y=w639) -> (x < y?=w638:bool)
        n235 = Increment(x=w637) -> (x+1=w641:i16)
        n236 = Not(x=w638) -> (.not. x?=w643:bool)
        n237 = Select(t=i16 0, s=w643, f=w641) -> (s? t:f=w640:i16)
        n238 = xnode "FPGA I/O Node"("Connector0/AO7"=w637) -> ()  [unwired: 1 in, 1 out]
        "Numeric" <- w637
      }
    }
  }
  n239 = while {
    stop <- FALSE stop-if-true
    n240 = xnode "FPGA I/O Node"() -> ("Connector0/AI0"=→"Connector0/AI0")  [unwired: 1 in, 1 out]
  }
  n241 = timed-loop {
    shift-right: [w647] -> _
    shift-left: u64 0 -> [w650]
    shift-right: [w649] -> _
    shift-left: TRUE -> [w648]
    timing: w8 -> [_]
    timing-out: [_] -> w7
    tunnel: [w649] -> _
    stop <- _ stop-if-true
    n242 = case shown="False" "square wave  on?" {
      tunnel: w650 -> [w652 w656]
      tunnel: [w651 w660] -> w649
      tunnel: w648 -> [w651 w659]
      tunnel: [w652 w657] -> w647
      frame False {
      }
      frame True {
        n243 = local read "square wave period"() -> (w655:i32)
        n244 = xnode "FPGA I/O Node"("Connector1/DIO6"=w659) -> ()  [unwired: 1 in, 1 out]
        n245 = Less?(x=w656, y=w655) -> (x < y?=w653:bool)
        n246 = Not(x=w653) -> (.not. x?=w654:bool)
        n247 = Increment(x=w656) -> (x+1=w662:u64)
        n248 = Not(x=w659) -> (.not. x?=w661:bool)
        n249 = Select(t=i16 0, s=w654, f=w662) -> (s? t:f=w657:u64)
        n250 = Greater Or Equal?(x=w657, y=w655) -> (x >= y?=w658:bool)
        n251 = Select(t=w661, s=w658, f=w659) -> (s? t:f=w660:bool)
      }
    }
  }
  n252 = node-c288(w7) -> ()
